vi "CheckSum.vi"(10 "DataIn":u8[](array[numeric]) format="%x") -> (1 "CheckSum":u8 format="%x", 2 "DataOut":u8[](array[numeric]) format="%x")   [LabVIEW 2013]
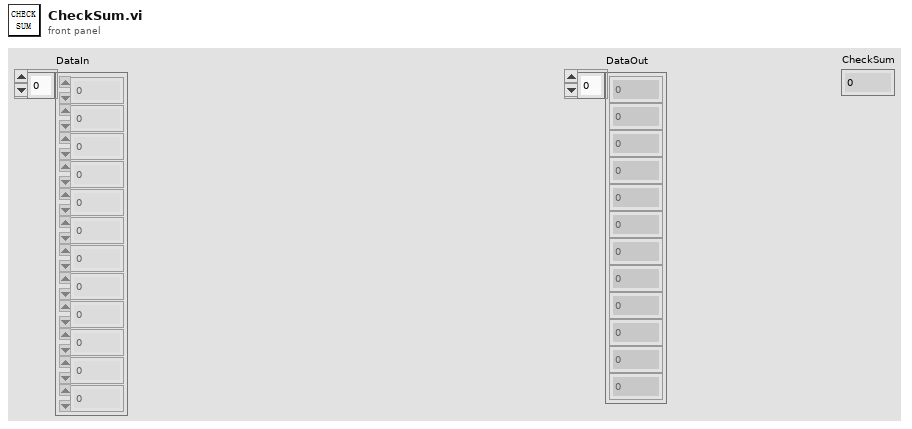
[diagram p1: front panel]
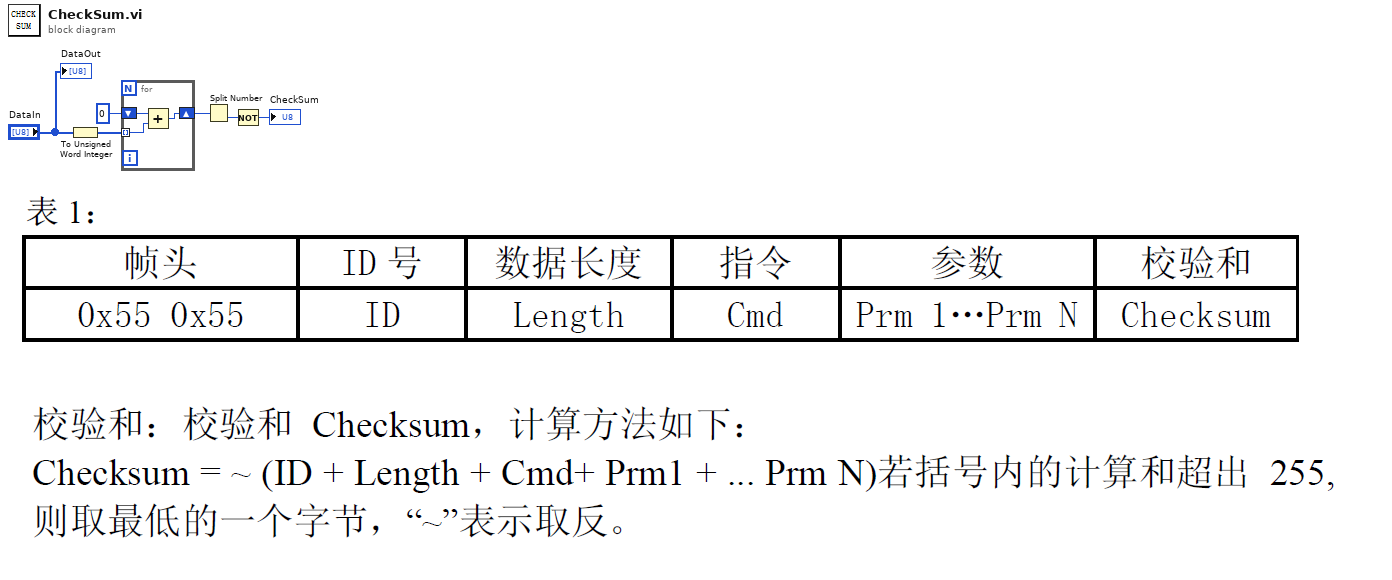
[diagram p0: block diagram]
diagram:
  n1 = To Unsigned Word Integer(number="DataIn") -> (unsigned 16bit integer=w5:u16[])
  n2 = for {
    shift-right: [w7] -> w4
    shift-left: u16 0 -> [w9]
    tunnel: w5 -> [w8] mode=indexing
    n3 = Add(x=w9, y=w8) -> (x+y=w7:u16)
  }
  n4 = Split Number(x=w4) -> (lo(x)=w3:u8)  [unwired: 1 out]
  n5 = Not(x=w3) -> (.not. x?=→"CheckSum":u8)
  "DataOut" <- "DataIn"
